vi "Gear Side Vision Processing.vi"(8 "error in (no error) 2":errorcluster, 11 "Image Size 2":T1=enum."320x240") -> (0 "Calibration error 2":errorcluster)   [LabVIEW 2016]
uses:
  <vilib>/Rock Robotics/WPI/Camera/WPI_CameraImageSize.ctl
  <vilib>/Rock Robotics/WPI/Camera/WPI_CameraFrameRate.ctl
  <vilib>/Rock Robotics/WPI/Camera/WPI_CameraWhite Balance Values.ctl
  <vilib>/Rock Robotics/WPI/Camera/WPI_CameraExposure Values.ctl
  Robot Global Data.vi
  <vilib>/Rock Robotics/Network Tables/NT Write Number.vi
  <vilib>/vision/NI_Vision_Development_Module.lvlib
  2039lib.lvlib
panel:
  out "Enable Vision":bool
  in  "LED Color 2":T2={"Hue"={107.81818389892578, 139.81818389892578}, "Sat"={176.07142857142858, 255.0}, "Val"={40.53571428571429, 255.0}} {"Hue" scale=0.0..255.0 scale format="%#_3g"}
  out "Qualified Particles 2":i32
  in  "Color Mode 2":u16(ring)=3 items=["RGB", "HSL", "HSV", "HSI"]
  in  "Use Calibration 2":bool=TRUE
  in  "Line Border 2":cluster{"Top":dbl, "Bottom":dbl}={"Top"=6.0, "Bottom"=1.0}
  in  "Display Mask 2":bool
  out "Mask 2":T3(plugin-control)
  in  "Count Objects Settings":T4={"Objects"=0, "Threshold"=128, "Reject Border"=TRUE, "Fill Holes"=FALSE, "Min Object Size"=TRUE, "Min Size"=30, "Max Object Size"=FALSE, "Max Size"=100, "Show Search Area"=FALSE, "Show Center"=TRUE, "Show Bounding Box"=TRUE} {"Objects" items=["Bright Objects", "Dark Objects"]; "Threshold" min=1 max=999999999 step=1; "Max Size" min=1 max=999999999 step=1; "Min Size" min=1 max=999999999 step=1}
  out "Overlaid Original":T3(plugin-control)
  out "loop ms 2":u32
  # "Legend:\n    Rectangle\n       Green - Good target, distance ft\n       Red - Bad target\n    Orange Text - Score in %"
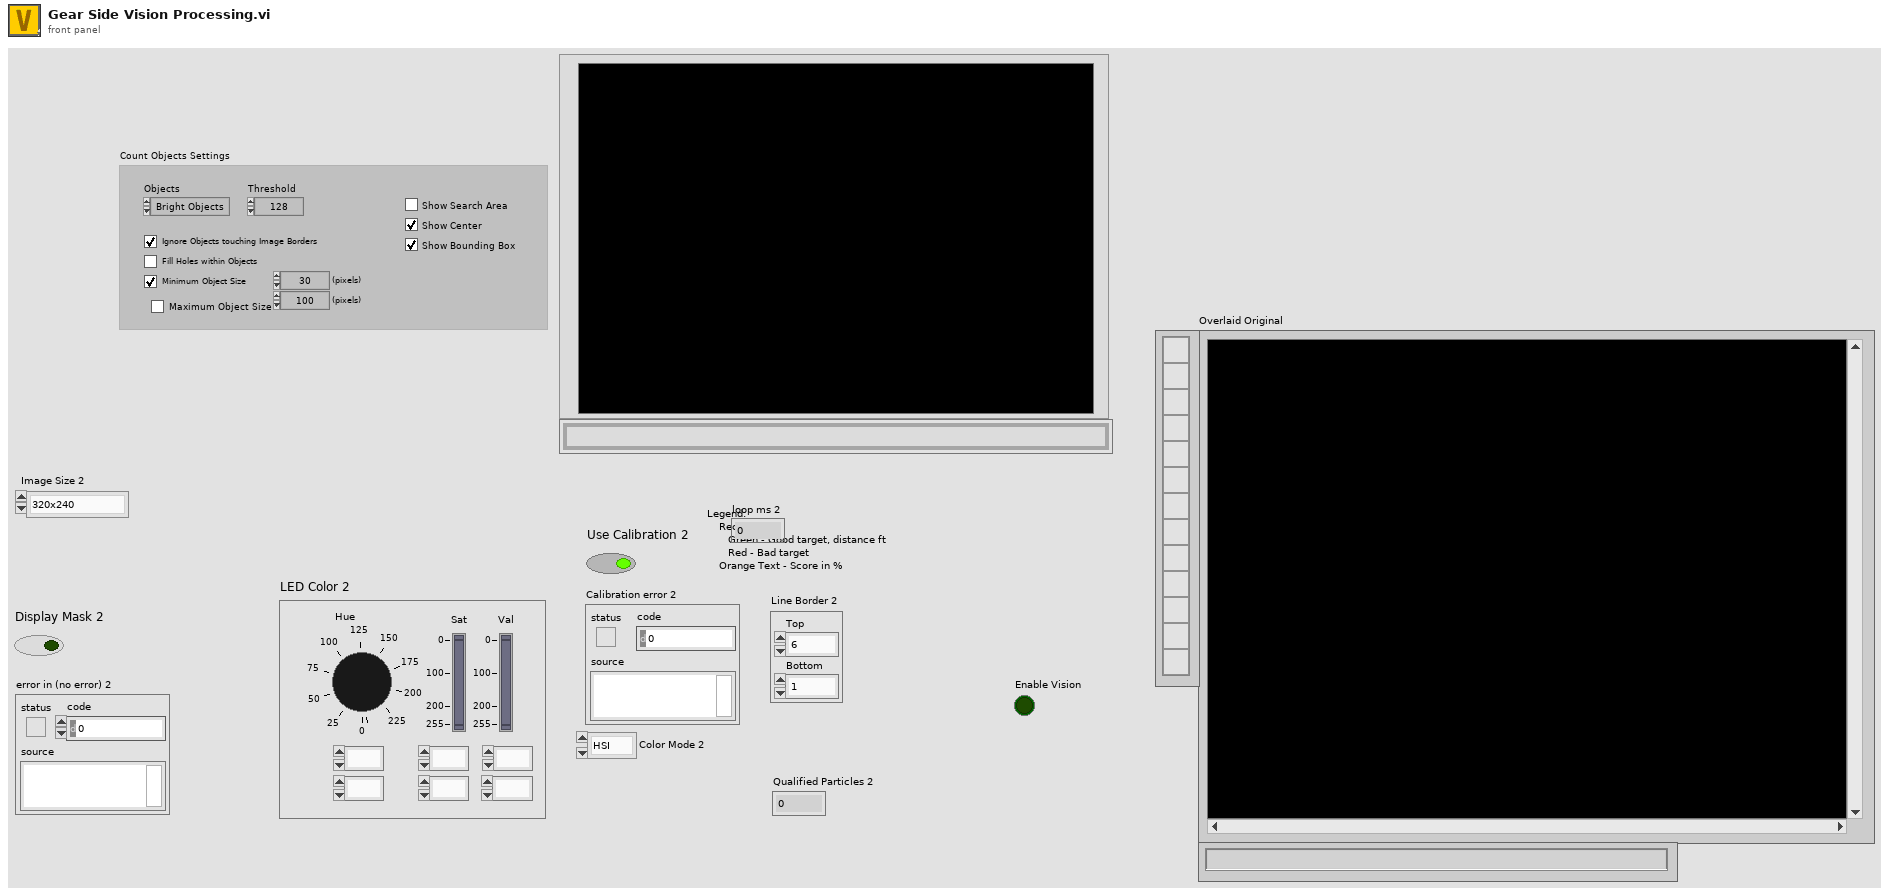
[diagram p1: front panel]
types:
  T1 = typedef "WPI_CameraImageSize.ctl" = enum16{"640x480", "320x240", "160x120", "Custom"}
  T2 = cluster{"Hue":cluster{dbl, dbl}, "Sat":cluster{dbl, dbl}, "Val":cluster{dbl, dbl}}
  T3 = typedef "IMAQ Image.ctl" = refnum<image>
  T4 = cluster{"Objects":u16, "Threshold":i32, "Reject Border":bool, "Fill Holes":bool, "Min Object Size":bool, "Min Size":i32, "Max Object Size":bool, "Max Size":i32, "Show Search Area":bool, "Show Center":bool, "Show Bounding Box":bool}
  T5 = typedef "WPI_CameraFrameRate.ctl" = u32
  T6 = typedef "WPI_CameraExposure Values.ctl" = enum16{"Auto", "Flicker-free 50 Hz", "Flicker-free 60 Hz", "Hold current", "Custom"}
  T7 = typedef "WPI_CameraWhite Balance Values.ctl" = enum16{"Auto", "Fixed indoor", "Fixed outdoor 1", "Fixed outdoor 2", "Fixed fluorescent 1", "Fixed fluorescent 2", "Hold current", "Custom"}
  T8 = typedef "Image Type" = u32
  T9 = typedef "WPI_CameraDevRef.ctl" = cluster{"Camera Address":string, "CameraStatus":errorcluster}
  T10 = cluster{"Object Center":cluster{"X":sgl, "Y":sgl}, "Bounding Box":cluster{"X Left":i32, "Y Top":i32, "X Right":i32, "Y Bottom":i32}, "Area":sgl, "Orientation":sgl, "Aspect Ratio":sgl, "Nb Holes":i32}[]
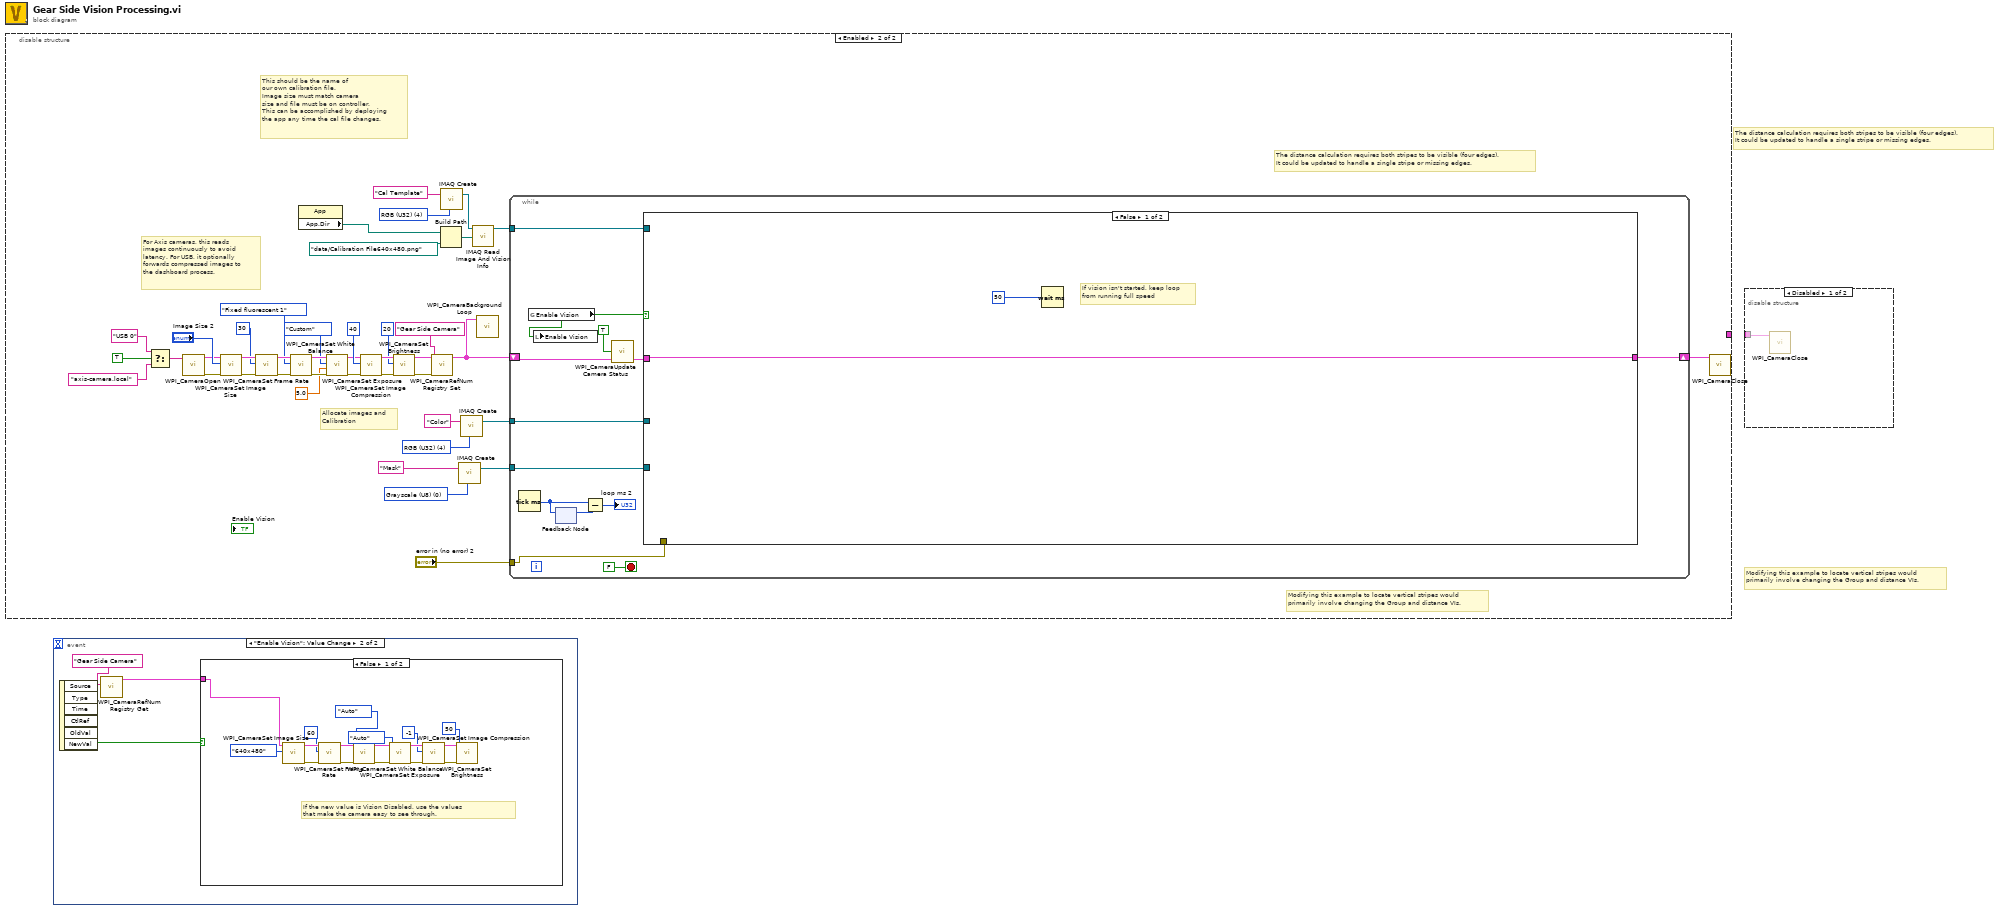
[diagram p0: block diagram]
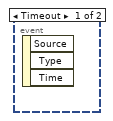
[diagram p2: hidden frame]
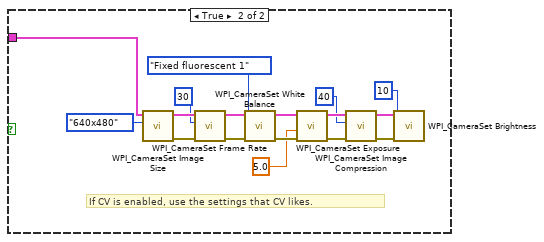
[diagram p3: hidden frame]
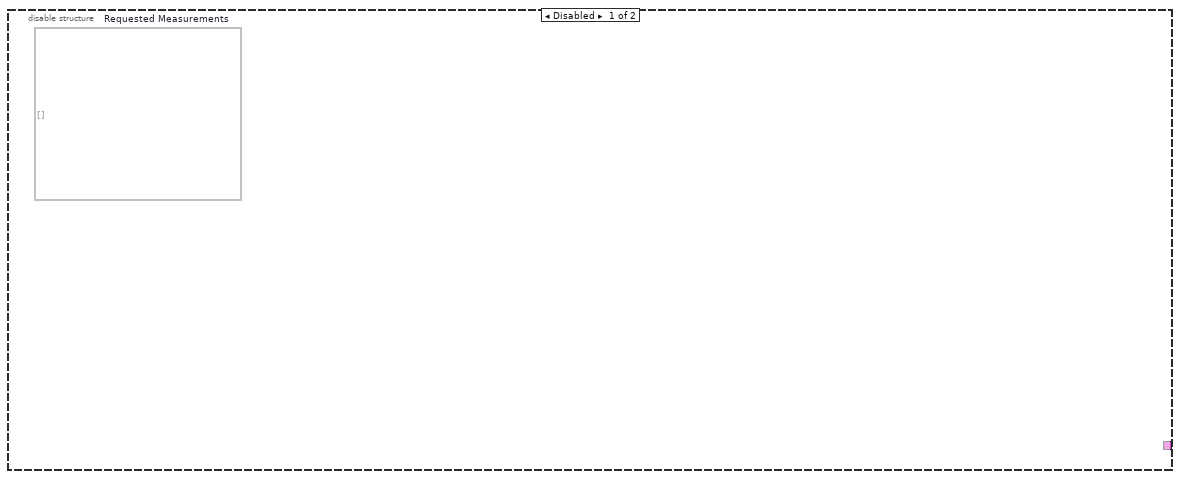
[diagram p5: hidden frame]
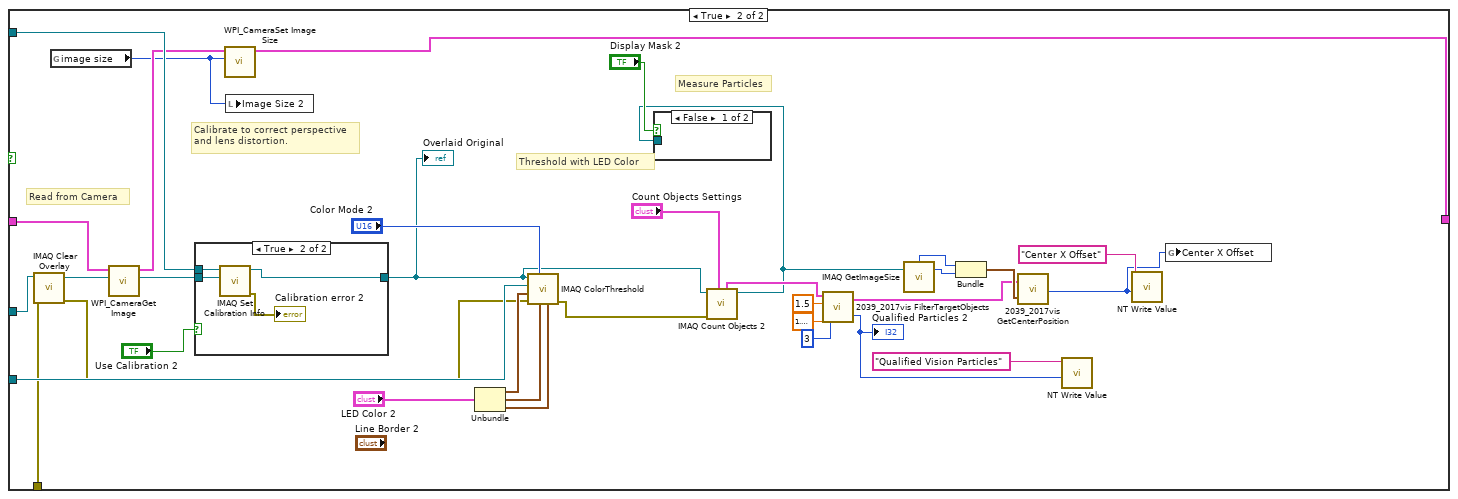
[diagram p6: hidden frame]
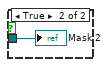
[diagram p7: hidden frame]
diagram:
  # "Modifying this example to locate vertical stripes would\nprimarily involve changing the Group and distance VIs."
  # "The distance calculation requires both stripes to be visible (four edges).\nIt could be updated to handle a single stripe or missing edges."
  n1 = disable-structure shown="Enabled" {
    disable-tunnel: _ -> [w1 _]
    frame Disabled {
      (unwired) void[] []  # Requested Measurements
    }
    frame Enabled {
      w37 = T8 4 items=["Grayscale (U8)", "Grayscale (I16)", "Grayscale (SGL)", "Complex (CSG)", "RGB (U32)", "HSL (U32)", "RGB (U64)", "Grayscale (U16)"] ("Image Type")
      w41 = T8 0 items=["Grayscale (U8)", "Grayscale (I16)", "Grayscale (SGL)", "Complex (CSG)", "RGB (U32)", "HSL (U32)", "RGB (U64)", "Grayscale (U16)"] ("Image Type")
      w42 = T8 4 items=["Grayscale (U8)", "Grayscale (I16)", "Grayscale (SGL)", "Complex (CSG)", "RGB (U32)", "HSL (U32)", "RGB (U64)", "Grayscale (U16)"] ("Image Type")
      # "This should be the name of \nour own calibration file.\nImage size must match camera\nsize and file must be on controller.\nThis can be accomplished by deploying\nthe app any time the cal file changes."
      # "For Axis cameras, this reads\nimages continuously to avoid\nlatency. For USB, it optionally\nforwards compressed images to\nthe dashboard process."
      # "Modifying this example to locate vertical stripes would\nprimarily involve changing the Group and distance VIs."
      # "The distance calculation requires both stripes to be visible (four edges).\nIt could be updated to handle a single stripe or missing edges."
      # "Allocate images and\nCalibration"
      n2 = Select(t="USB 0" ("format string"), s=TRUE ("dot notation? (F)"), f="axis-camera.local" ("format string")) -> (s? t:f=w8:string)
      n3 = call <vilib>:"WPI_CameraOpen.vi"("Camera Address"=w8) -> ("error out"=w20:errorcluster, "CameraDevRef"=w21:T9)  [unwired: 1 in, 8 out]
      n4 = call <vilib>:"WPI_CameraSet Image Size.vi"("error in (no error)"=w20, "Image Size"="Image Size 2", "CameraDevRef"=w21) -> ("error out"=w19:errorcluster, "CameraDevRef Out"=w22:T9)  [unwired: 1 in, 6 out]
      n5 = call <vilib>:"WPI_CameraSet Frame Rate.vi"("error in (no error)"=w19, "Frame Rate (fps)"=T5 30, "CameraDevRef"=w22) -> ("error out"=w18:errorcluster, "CameraDevRef Out"=w24:T9)  [unwired: 7 out]
      n6 = call <vilib>:"WPI_CameraSet White Balance.vi"("error in (no error)"=w18, "White Balance"=WPI_CameraWhite_Balance_Values."Fixed fluorescent 1", "CameraDevRef"=w24) -> ("error out"=w17:errorcluster, "CameraDevRef Out"=w23:T9)  [unwired: 1 in, 6 out]
      n7 = property class="App"() -> ("App.Dir"=w3:path)  [unwired: 2 in, 2 out]
      n8 = call <vilib>:"WPI_CameraSet Exposure.vi"("error in (no error)"=w17, "Exposure (%)"=5.0, "Exposure"=WPI_CameraExposure_Values."Custom", "CameraDevRef"=w23) -> ("error out"=w16:errorcluster, "CameraDevRef Out"=w26:T9)  [unwired: 6 out]
      n9 = call <vilib>:"WPI_CameraSet Image Compression.vi"("error in (no error)"=w16, "Compression"=40, "CameraDevRef"=w26) -> ("error out"=w15:errorcluster, "CameraDevRef Out"=w25:T9)  [unwired: 7 out]
      n10 = call <vilib>:"WPI_CameraSet Brightness.vi"("error in (no error)"=w15, "Brightness"=20, "CameraDevRef"=w25) -> ("error out"=w14:errorcluster, "CameraDevRef Out"=w31:T9)  [unwired: 7 out]
      n11 = call <vilib>:"WPI_CameraRefNum Registry Set.vi"("error in (no error)"=w14, "refnum name"="Gear Side Camera", "CameraDevRef"=w31) -> ("CameraDevRef"=w7:T9)  [unwired: 1 in, 7 out]
      n12 = Build Path(base path=w3, name or relative path=path "data/Calibration File640x480.png" ("Folder Location")) -> (appended path=w33:path)
      n13 = call "IMAQ Create"("Image Name"="Cal Template", "Image Type"=w37) -> ("New Image"=w35:T3)  [unwired: 2 in, 2 out]
      n14 = call "IMAQ Create"("Image Name"="Mask", "Image Type"=w41) -> ("New Image"=w39:T3)  [unwired: 2 in, 2 out]
      n15 = call "IMAQ Create"("Image Name"="Color", "Image Type"=w42) -> ("New Image"=w38:T3)  [unwired: 2 in, 2 out]
      n16 = call "IMAQ Read Image And Vision Info"("File Path"=w33, "Image"=w35) -> ("Image Out"=w34:T3)  [unwired: 7 in, 2 out]
      n17 = call <vilib>:"WPI_CameraBackground Loop.vi"("CameraDevRef"=w7) -> ()  [unwired: 11 in]
      n18 = while {
        tunnel: w38 -> [w53]
        tunnel: w39 -> [w55]
        tunnel: w34 -> [w54]
        shift-right: [w52] -> w6
        shift-left: w7 -> [w51]
        tunnel: "error in (no error) 2" -> [w46]
        stop <- FALSE stop-if-true
        n19 = Tick Count (ms)() -> (millisecond timer value=w48:u32)
        n20 = global read "Robot Global Data.vi" "Enable Vision"() -> (w45:bool)
        n21 = local write "Enable Vision"(w45) -> ()
        n22 = feedback-in #1(w48) -> ()
        n23 = feedback #1() -> (w49:u32)  [unwired: 1 in]
        n24 = Subtract(x=w48, y=w49) -> (x-y=→"loop ms 2":u32)
        n25 = call <vilib>:"WPI_CameraUpdate Camera Status.vi"("CameraDevRef In"=w51, "Enable Vision"=TRUE) -> ("CameraDevRef Out"=w50:T9)  [unwired: 3 in]
        n26 = case shown="False" w45 {
          tunnel: w55 -> [_ w92]
          tunnel: w54 -> [_ w86]
          tunnel: w50 -> [w58 w84]
          tunnel: w53 -> [_ w77]
          tunnel: [w58 w78] -> w52
          tunnel: w46 -> [_ w73]
          frame False {
            # "If vision isn't started, keep loop\nfrom running full speed"
            n27 = Wait (ms)(milliseconds to wait=u32 50) -> ()  [unwired: 1 out]
          }
          frame True {
            # "Read from Camera"
            # "Calibrate to correct perspective\nand lens distortion."
            # "Measure Particles"
            # "Threshold with LED Color"
            n28 = call "IMAQ Clear Overlay"("error in (no error)"=w73, "Image"=w77) -> ("error out"=w74:errorcluster, "Image Out"=w76:T3)  [unwired: 8 in]
            n29 = global read "Robot Global Data.vi" "image size"() -> (w80:T1)
            n30 = call <vilib>:"WPI_CameraGet Image.vi"("Image"=w76, "CameraDevRef"=w84) -> ("Image Out"=w83:T3, "CameraDevRef Out"=w81:T9)  [unwired: 7 in, 1 out]
            n31 = case shown="True" "Use Calibration 2" {
              tunnel: [w94 w98] -> w59
              tunnel: w83 -> [w94 w97]
              tunnel: w86 -> [_ w96]
              frame False {
              }
              frame True {
                n32 = call "IMAQ Set Calibration Info"("Image Dst"=w97, "Image Src"=w96) -> ("error out"=→"Calibration error 2":errorcluster, "Calibrated Image"=w98:T3)  [unwired: 8 in]
              }
            }
            "Overlaid Original" <- w59
            n33 = call <vilib>:"WPI_CameraSet Image Size.vi"("Image Size"=w80, "CameraDevRef"=w81) -> ("CameraDevRef Out"=w78:T9)  [unwired: 2 in, 7 out]
            n34 = local write "Image Size 2"(w80) -> ()
            n35 = Unbundle("LED Color 2") -> ("Hue"=w91:cluster{dbl, dbl}, "Sat"=w90:cluster{dbl, dbl}, "Val"=w89:cluster{dbl, dbl})
            n36 = call "IMAQ ColorThreshold"("Blue or Luma or Val or Inten Range"=w89, "Green or Sat Range"=w90, "Color Mode"="Color Mode 2", "error in (no error)"=w74, "Red or Hue Range"=w91, "Image Dst"=w92, "Image Src"=w59) -> ("error out"=w75:errorcluster)  [unwired: 3 in, 1 out]
            n37 = call "IMAQ Count Objects 2"("Settings"="Count Objects Settings", "error in (no error)"=w75, "Image"=w59) -> ("Image Out"=w68:T3, "Objects"=w72:T10)  [unwired: 4 in, 3 out]
            n38 = case shown="False" "Display Mask 2" {
              tunnel: w68 -> [_ w93]
              frame False {
              }
              frame True {
                "Mask 2" <- w93
              }
            }
            n39 = call "2039_2017vis FilterTargetObjects.vi"("Holes Limit"=3, "Lower Aspect Ratio Limit"=sgl 1.3, "Upper Aspect Ratio Limit"=sgl 1.5, "Objects"=w72) -> ("Number of Qualified Objects"=w63:i32, "Qualified Objects"=w64:T10)
            "Qualified Particles 2" <- w63
            n40 = call "IMAQ GetImageSize"("Image"=w68) -> ("Y Resolution"=w66:i32, "X Resolution"=w67:i32)  [unwired: 3 in, 1 out]
            n41 = Bundle("X Resolution"=w67, "Y Resolution"=w66) -> (w65:cluster{"X Resolution":i32, "Y Resolution":i32})  [unwired: 1 in]
            n42 = call "2039_2017vis GetCenterPosition.vi"("Image Size"=w65, "Objects"=w64) -> ("Center X Offset"=w60:i32)
            n43 = call-poly <vilib>:"NT Write Value.vi"("Numeric"=w63, "Name"="Qualified Vision Particles") -> ()  [unwired: 9 in, 1 out]
            n44 = call-poly <vilib>:"NT Write Value.vi"("Numeric"=w60, "Name"="Center X Offset") -> ()  [unwired: 9 in, 1 out]
            n45 = global write "Robot Global Data.vi" "Center X Offset"(w60) -> ()
          }
        }
      }
      n46 = call <vilib>:"WPI_CameraClose.vi"("CameraDevRef"=w6) -> ()  [unwired: 1 in, 10 out]
    }
  }
  n47 = event shown="[1] \"Enable Vision\": Value Change" {
    selector: _ -> [_ _]
    dyn-events: _ -> [_ _]
    timeout: _ -> [_ _]
    event Timeout {
      n48 = event-data() -> ()  [unwired: 1 in, 3 out]
    }
    event "Enable Vision": Value Change {
      n49 = event-data() -> ("NewVal"=w101:bool)  [unwired: 1 in, 5 out]
      n50 = call <vilib>:"WPI_CameraRefNum Registry Get.vi"("refnum name"="Gear Side Camera") -> ("CameraDevRef"=w99:T9)  [unwired: 9 in, 1 out]
      n51 = case shown="False" w101 {
        tunnel: w99 -> [w103 w124]
        frame False {
          # "If the new value is Vision Disabled, use the values\nthat make the camera easy to see through."
          n52 = call <vilib>:"WPI_CameraSet Image Size.vi"("Image Size"=WPI_CameraImageSize."640x480", "CameraDevRef"=w103) -> ("error out"=w113:errorcluster, "CameraDevRef Out"=w114:T9)  [unwired: 2 in, 6 out]
          n53 = call <vilib>:"WPI_CameraSet Frame Rate.vi"("error in (no error)"=w113, "Frame Rate (fps)"=T5 60, "CameraDevRef"=w114) -> ("error out"=w112:errorcluster, "CameraDevRef Out"=w116:T9)  [unwired: 7 out]
          n54 = call <vilib>:"WPI_CameraSet White Balance.vi"("error in (no error)"=w112, "White Balance"=WPI_CameraWhite_Balance_Values."Auto", "CameraDevRef"=w116) -> ("error out"=w111:errorcluster, "CameraDevRef Out"=w115:T9)  [unwired: 1 in, 6 out]
          n55 = call <vilib>:"WPI_CameraSet Exposure.vi"("error in (no error)"=w111, "Exposure"=WPI_CameraExposure_Values."Auto", "CameraDevRef"=w115) -> ("error out"=w110:errorcluster, "CameraDevRef Out"=w118:T9)  [unwired: 1 in, 6 out]
          n56 = call <vilib>:"WPI_CameraSet Image Compression.vi"("error in (no error)"=w110, "Compression"=-1, "CameraDevRef"=w118) -> ("error out"=w109:errorcluster, "CameraDevRef Out"=w117:T9)  [unwired: 7 out]
          n57 = call <vilib>:"WPI_CameraSet Brightness.vi"("error in (no error)"=w109, "Brightness"=50, "CameraDevRef"=w117) -> ()  [unwired: 9 out]
        }
        frame True {
          # "If CV is enabled, use the settings that CV likes."
          n58 = call <vilib>:"WPI_CameraSet Image Size.vi"("Image Size"=WPI_CameraImageSize."640x480", "CameraDevRef"=w124) -> ("error out"=w130:errorcluster, "CameraDevRef Out"=w131:T9)  [unwired: 2 in, 6 out]
          n59 = call <vilib>:"WPI_CameraSet Frame Rate.vi"("error in (no error)"=w130, "Frame Rate (fps)"=T5 30, "CameraDevRef"=w131) -> ("error out"=w129:errorcluster, "CameraDevRef Out"=w133:T9)  [unwired: 7 out]
          n60 = call <vilib>:"WPI_CameraSet White Balance.vi"("error in (no error)"=w129, "White Balance"=WPI_CameraWhite_Balance_Values."Fixed fluorescent 1", "CameraDevRef"=w133) -> ("error out"=w128:errorcluster, "CameraDevRef Out"=w132:T9)  [unwired: 1 in, 6 out]
          n61 = call <vilib>:"WPI_CameraSet Exposure.vi"("error in (no error)"=w128, "Exposure (%)"=5.0, "CameraDevRef"=w132) -> ("error out"=w127:errorcluster, "CameraDevRef Out"=w135:T9)  [unwired: 1 in, 6 out]
          n62 = call <vilib>:"WPI_CameraSet Image Compression.vi"("error in (no error)"=w127, "Compression"=40, "CameraDevRef"=w135) -> ("error out"=w126:errorcluster, "CameraDevRef Out"=w134:T9)  [unwired: 7 out]
          n63 = call <vilib>:"WPI_CameraSet Brightness.vi"("error in (no error)"=w126, "Brightness"=10, "CameraDevRef"=w134) -> ()  [unwired: 9 out]
        }
      }
    }
  }
  n64 = disable-structure shown="Disabled" {
    disable-tunnel: _ -> [w136 _]
    frame Disabled {
      n65 = call <vilib>:"WPI_CameraClose.vi"("CameraDevRef"=w136) -> ()  [unwired: 1 in, 10 out]
    }
    frame Enabled {
    }
  }
